vi "dfd_Classical FIR Filter Design Params Validation.vi"(6 "fs [Hz]":dbl=1.0 format="%.2f", 7 "filter type":T1(ring), 8 "error in (no error)":errorcluster, 9 "low cutoff freq: fl":dbl, 10 "high cutoff freq: fh":dbl, 11 "order":i32) -> (0 "error out":errorcluster)   [LabVIEW 2017, in "NI_DigFilter_Design.lvlib"]
uses:
  <vilib>/addons/Digital Filter Design/NI_DigFilter_Design.lvlib
  <vilib>/addons/Digital Filter Design/_Misc.llb/dfd_Error Handlers (Multiple).vi
  <vilib>/addons/Digital Filter Design/NI_DigFilterLicensed.lvlib
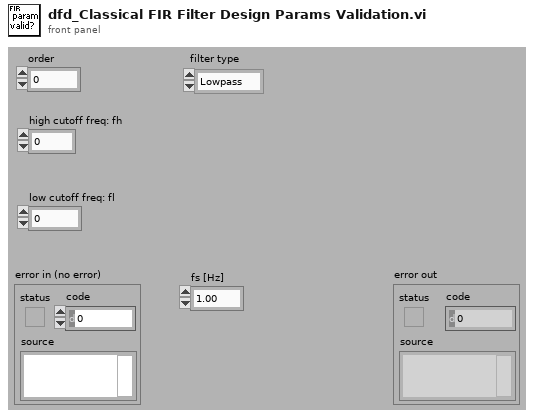
[diagram p1: front panel]
types:
  T1 = enum16{"Lowpass", "Highpass", "Bandpass", "Bandstop"}
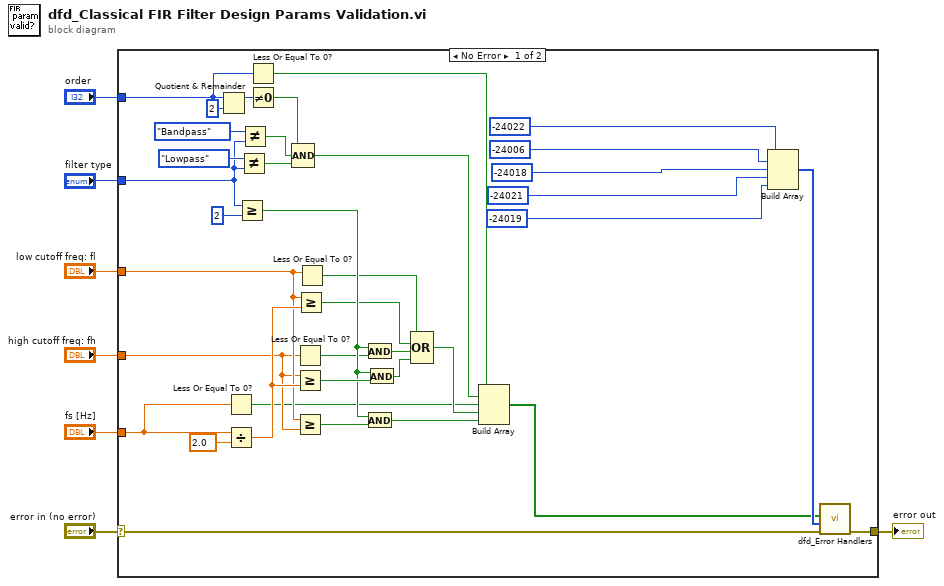
[diagram p0: block diagram]
diagram:
  n1 = case shown="No Error" "error in (no error)" {
    selector: "error in (no error)" -> [w29 w45]
    tunnel: "filter type" -> [w22 _]
    tunnel: "fs [Hz]" -> [w44 _]
    tunnel: [w43 w45] -> w5
    tunnel: "order" -> [w42 _]
    tunnel: "low cutoff freq: fl" -> [w27 _]
    tunnel: "high cutoff freq: fh" -> [w19 _]
    frame No Error {
      n2 = Quotient & Remainder(x=w42, y=2) -> (x-y*floor(x/y)=w40:i32)  [unwired: 1 out]
      n3 = Less Or Equal To 0?(x=w44) -> (x <= 0?=w11:bool)
      n4 = Divide(x=w44, y=2.0) -> (x/y=w28:dbl)
      n5 = Greater Or Equal?(x=w22, y=2) -> (x >= y?=w17:bool)
      n6 = Not Equal?(x=T1."Lowpass", y=w22) -> (x != y?=w21:bool)
      n7 = Not Equal?(x=T1."Bandpass", y=w22) -> (x != y?=w20:bool)
      n8 = Less Or Equal To 0?(x=w42) -> (x <= 0?=w36:bool)
      n9 = Not Equal To 0?(x=w40) -> (x != 0?=w37:bool)
      n10 = Compound Arithmetic op=AND(w37, w20, w21) -> (w12:bool)
      n11 = Less Or Equal To 0?(x=w19) -> (x <= 0?=w16:bool)
      n12 = Greater Or Equal?(x=w19, y=w28) -> (x >= y?=w18:bool)
      n13 = Greater Or Equal?(x=w27, y=w19) -> (x >= y?=w31:bool)
      n14 = Greater Or Equal?(x=w27, y=w28) -> (x >= y?=w14:bool)
      n15 = Less Or Equal To 0?(x=w27) -> (x <= 0?=w13:bool)
      n16 = And(x=w17, y=w16) -> (x .and. y?=w15:bool)
      n17 = And(x=w17, y=w31) -> (x .and. y?=w10:bool)
      n18 = And(x=w17, y=w18) -> (x .and. y?=w26:bool)
      n19 = Compound Arithmetic op=OR(w13, w14, w15, w26) -> (w25:bool)
      n20 = Build Array(w36, w12, w11, w25, w10) -> (w32:bool[])
      n21 = Build Array(-24022 ("ERR_ORDER_LE_ZERO"), -24006 ("ERR_TYPE_II_HIGHPASS"), -24018 ("ERR_FS_LE_ZERO"), -24021 ("ERR_FREQ_RANGE_WRONG"), -24019 ("ERR_FREQ_NOT_ASCENDING")) -> (w33:i32[])
      n22 = call-poly <vilib>:"dfd_Error Handlers.vi"("error in (no error)"=w29, "error sources"=w33, "condition failed?"=w32) -> ("error out"=w43:errorcluster)  [unwired: 8 out]
    }
    frame Error {
    }
  }
  "error out" <- w5
